vi "thread.vi"(0 "HGF_ThreadWorker":refnum<class "HGF_ThreadWorker.lvclass">, 1 "HGF_ThreadPool_Reference":refnum<class "HGF_Reference.lvclass">, 5 "error in (no error)":errorcluster) -> (19 "error out":errorcluster)   [LabVIEW 2014, in "HGF_BaseClasses.lvlib" / "HGF_ThreadWorker.lvclass"]
doc: "This is the thread started from the HGF_ThreadPool.\n\n<b>Attention:</b> This VI is reentrant and sharing sources."
uses:
  HGF_ThreadWorker.lvclass
  HGF_ThreadPool/HGF_ThreadPool.lvclass
  HGF_Reference/HGF_Reference.lvclass
  HGF_ThreadTask/HGF_ThreadTask.lvclass
  HGF_Auxiliary/HGF_Auxiliary.lvlib
  HGF_Event/HGF_Event.lvclass
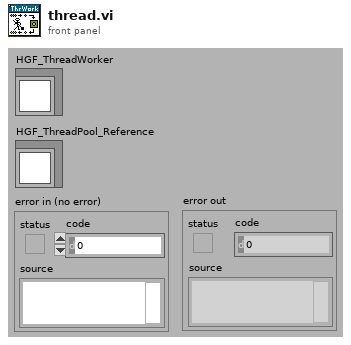
[diagram p1: front panel]
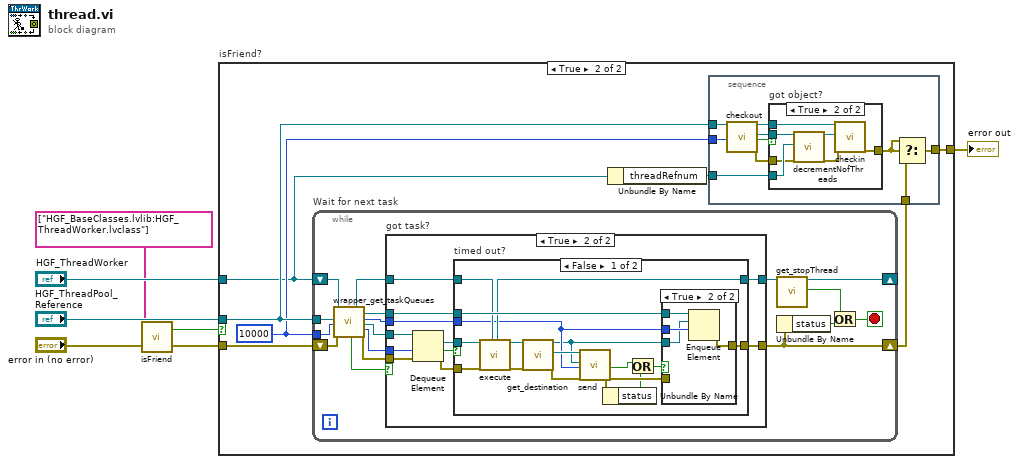
[diagram p0: block diagram]
diagram:
  n1 = call "isFriend.vi"("error in (no error)"="error in (no error)", "Friends"=string[] ["HGF_BaseClasses.lvlib:HGF_ThreadWorker.lvclass"]) -> ("error out"=w3:errorcluster, "isFriend?"=w1:bool)
  n2 = case "isFriend?" shown="True" w1 {
    tunnel: "HGF_ThreadPool_Reference" -> [_ w15]
    tunnel: [w8 w11] -> w6
    tunnel: "HGF_ThreadWorker" -> [_ w10]
    tunnel: w3 -> [w8 w9]
    frame False {
    }
    frame True {
      w13 = 10000 ("timeout in ms (-1)")
      n3 = while "Wait for next task" {
        shift-right: [w34] -> _
        shift-left: w10 -> [w47]
        tunnel: w15 -> [w45]
        shift-right: [w49] -> w14
        shift-left: w9 -> [w43]
        tunnel: w13 -> [w44]
        stop <- w50 stop-if-true
        n4 = call "wrapper_get_taskQueues.vi"("HGF_ThreadWorker in"=w47, "HGF_ThreadPool_Reference"=w45, "timeout in ms (-1)"=w44, "error in (no error)"=w43) -> ("got object?"=w41:bool, "HGF_ThreadWorker out"=w46:refnum<class "HGF_ThreadWorker.lvclass">, "taskQueue out"=w40:refnum<queue>, "timeoutTaskQueueOut"=w39:i32, "taskQueue in"=w38:refnum<queue>, "timeoutTaskQueueIn"=w37:i32, "error out"=w42:errorcluster)  [unwired: 9 in]
        n5 = case "got task?" shown="True" w41 {
          tunnel: w42 -> [w51 w63]
          tunnel: w40 -> [_ w62]
          tunnel: w38 -> [_ w61]
          tunnel: w46 -> [w52 w57]
          tunnel: w37 -> [_ w60]
          tunnel: w39 -> [_ w59]
          tunnel: [w52 w53] -> w35
          tunnel: [w51 w58] -> w49
          frame False {
          }
          frame True {
            n6 = Dequeue Element(queue=w61, timeout in ms (-1)=w60, error in (no error)=w63) -> (element=w56:refnum<class "HGF_ThreadTask.lvclass">, timed out?=w54:bool, error out=w55:errorcluster)  [unwired: 1 out]
            n7 = case "timed out?" shown="False" w54 {
              tunnel: w62 -> [w79 _]
              tunnel: w59 -> [w69 _]
              tunnel: [w74 w86] -> w53
              tunnel: [w78 w85] -> w58
              tunnel: w57 -> [w75 w86]
              tunnel: w56 -> [w77 _]
              tunnel: w55 -> [w76 w85]
              frame False {
                n8 = call "execute.vi"("HGF_ThreadTask"=w77, "error in (no error)"=w76, "HGF_ThreadWorker"=w75) -> ("dup HGF_ThreadWorker"=w74:refnum<class "HGF_ThreadWorker.lvclass">, "dup HGF_ThreadTask"=w73:refnum<class "HGF_ThreadTask.lvclass">, "error out"=w72:errorcluster)  [unwired: 14 out]
                n9 = call "get_destination.vi"("HGF_ThreadTask"=w73, "error in (no error)"=w72) -> ("dup HGF_ThreadTask"=w68:refnum<class "HGF_ThreadTask.lvclass">, "destination"=w71:refnum<class "HGF_Event.lvclass">, "error out"=w70:errorcluster)  [unwired: 15 out]
                n10 = call-dynamic "send.vi"("HGF_Event"=w71, "Object"=w68, "timeout in ms (-1)"=w69, "error in (no error)"=w70) -> ("timed out?"=w66:bool, "error out"=w65:errorcluster)  [unwired: 1 in, 13 out]
                n11 = Unbundle By Name(w65) -> ("status"=w64:bool)
                n12 = Or(x=w66, y=w64) -> (x .or. y?=w67:bool)
                n13 = case shown="True" w67 {
                  tunnel: w79 -> [_ w84]
                  tunnel: [w80 w83] -> w78
                  tunnel: w69 -> [_ w82]
                  tunnel: w68 -> [_ w81]
                  tunnel: w65 -> [w80 _]
                  frame False {
                  }
                  frame True {
                    n14 = Enqueue Element(queue=w84, element=w81, timeout in ms (-1)=w82) -> (error out=w83:errorcluster)  [unwired: 1 in, 2 out]
                  }
                }
              }
              frame True {
              }
            }
          }
        }
        n15 = call "get_stopThread.vi"("HGF_ThreadWorker"=w35) -> ("dup HGF_ThreadWorker"=w34:refnum<class "HGF_ThreadWorker.lvclass">, "stopThread"=w36:bool)  [unwired: 1 in, 16 out]
        n16 = Unbundle By Name(w49) -> ("status"=w48:bool)
        n17 = Or(x=w36, y=w48) -> (x .or. y?=w50:bool)
      }
      n18 = Unbundle By Name(w10) -> ("threadRefnum"=w12:refnum<vi>)
      n19 = stacked-sequence {
        tunnel: w15 -> [w25]
        tunnel: w14 -> [w18]
        tunnel: w13 -> [w24]
        tunnel: w12 -> [w22]
        tunnel: [w17] -> w11
        frame #0 {
          n20 = call "checkout.vi"("HGF_ThreadPool_Reference"=w25, "timeout in ms (-1)"=w24) -> ("dup HGF_ThreadPool_Reference"=w20:refnum<class "HGF_Reference.lvclass">, "HGF_ThreadPool"=w23:refnum<class "HGF_ThreadPool.lvclass">, "got object?"=w19:bool, "error out"=w21:errorcluster)  [unwired: 1 in, 13 out]
          n21 = case "got object?" shown="True" w19 {
            tunnel: w23 -> [_ w33]
            tunnel: w22 -> [_ w32]
            tunnel: w21 -> [w26 w31]
            tunnel: w20 -> [_ w30]
            tunnel: [w26 w27] -> w16
            frame False {
            }
            frame True {
              n22 = call "decrementNofThreads.vi"("HGF_ThreadPool"=w33, "threadRef"=w32, "error in (no error)"=w31) -> ("dup HGF_ThreadPool"=w29:refnum<class "HGF_ThreadPool.lvclass">, "error out"=w28:errorcluster)  [unwired: 15 out]
              n23 = call "checkin.vi"("HGF_Reference"=w30, "Object"=w29, "error in (no error)"=w28) -> ("error out"=w27:errorcluster)  [unwired: 1 in, 15 out]
            }
          }
          n24 = Select(t=w16, s=w16, f=w18) -> (s? t:f=w17:errorcluster)
        }
      }
    }
  }
  "error out" <- w6
